vi "Remove Suffix.vi"(10 "Suffix":string, 11 "String":string) -> (2 "Suffix Missing?":bool, 3 "String out":string)   [LabVIEW 2015, in "E2E Tag Exchange editor node.lvclass"]
uses:
  E2E Tag Exchange editor node.lvclass
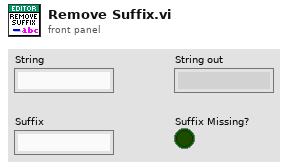
[diagram p1: front panel]
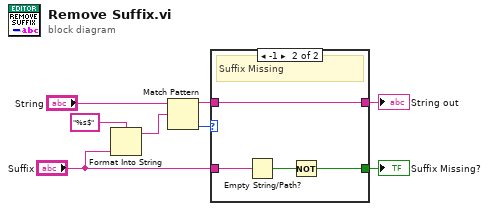
[diagram p0: block diagram]
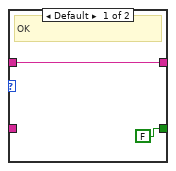
[diagram p2: hidden frame]
diagram:
  n1 = Format Into String(format string="%s$", "Suffix") -> (resulting string=w3:string)  [unwired: 2 in, 1 out]
  n2 = Match Pattern(string="String", regular expression=w3) -> (before substring=w5:string, offset past match=w6:i32)  [unwired: 1 in, 2 out]
  n3 = case shown="-1" w6 {
    tunnel: [FALSE w11] -> w8
    tunnel: w5 -> [w9 w14]
    tunnel: [w9 w14] -> w2
    tunnel: "Suffix" -> [_ w13]
    frame Default {
      # "OK"
    }
    frame -1 {
      # "Suffix Missing"
      n4 = Empty String/Path?(string/path=w13) -> (empty?=w12:bool)
      n5 = Not(x=w12) -> (.not. x?=w11:bool)
    }
  }
  "Suffix Missing?" <- w8
  "String out" <- w2
